vi "Create Rendezvous.vi"(8 "Error In":errorcluster, 10 "Treads":i32[](array[numeric]), 11 "Actor In":refnum<class "System Actor.lvclass">) -> (0 "Error Out":errorcluster, 3 "Actor Out":refnum<class "System Actor.lvclass">)   [LabVIEW 2024, in "System Actor.lvclass"]
uses:
  System Actor.lvclass
  System Actor.lvclass/System Actor.ctl
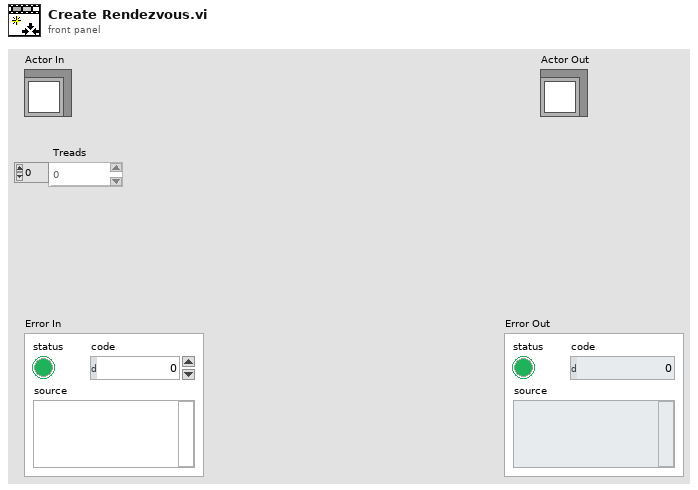
[diagram p1: front panel]
types:
  T1 = typedef "Rendezvous RefNum" = refnum<k1>
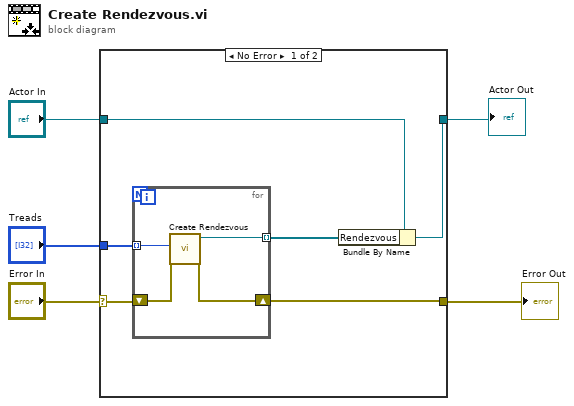
[diagram p0: block diagram]
diagram:
  n1 = case shown="No Error" "Error In" {
    selector: "Error In" -> [w11 w17]
    tunnel: [w9 w17] -> w4
    tunnel: [w6 w16] -> w2
    tunnel: "Actor In" -> [w8 w16]
    tunnel: "Treads" -> [w10 _]
    frame No Error {
      n2 = for {
        shift-right: [w13] -> w9
        shift-left: w11 -> [w14]
        tunnel: w10 -> [w15] mode=indexing
        tunnel: [w12] -> w7 mode=indexing
        n3 = call <vilib>:"Create Rendezvous.vi"("error in (no error)"=w14, "size (2)"=w15) -> ("error out"=w13:errorcluster, "rendezvous"=w12:T1)  [unwired: 3 in, 1 out]
      }
      n4 = Bundle By Name(cluster=w8, "Rendezvous"=w7) -> (w6:refnum<class "System Actor.lvclass">)
    }
    frame Error {
    }
  }
  "Actor Out" <- w2
  "Error Out" <- w4
